vi "myRIO_BRig_Host_parse_dataBlock__v4.vi"(10 "input_dataCurrent":u16[](array[numeric]), 11 "input_dataBlock":u16[][](array[numeric])) -> (0 "BlockR_T2R_avg":dbl caption="Trials2Reward", 1 "BlockR_BTPR_avg":dbl caption="BadTrialsPostReward", 2 "BlockL_BTPR_avg":dbl caption="BadTrialsPostReward" format="%#_3g", 3 "BlockL_T2R_avg":dbl caption="Trials2Reward" format="%#_3g", 4 "BlockR_BTPR_cur":u16 caption="BadTrialsPostReward", 5 "BlockL_BTPR_cur":u16 caption="BadTrialsPostReward", 6 "BlockR_T2R_cur":u16 caption="Trials2Reward", 7 "BlockL_T2R_cur":u16 caption="Trials2Reward")   [LabVIEW 2014]
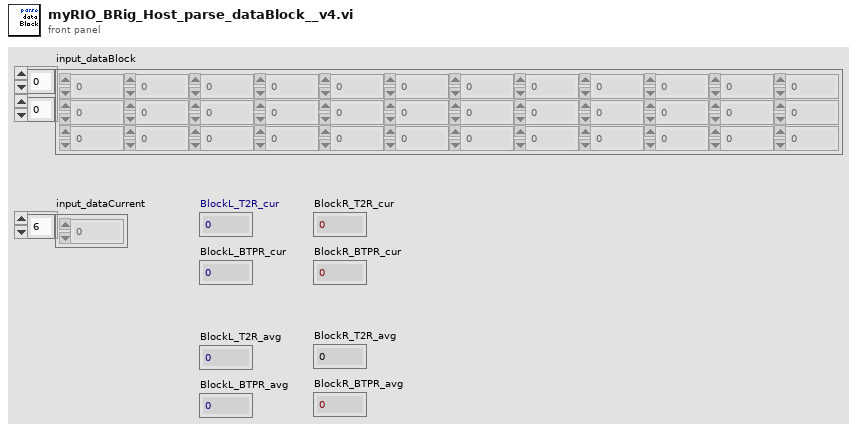
[diagram p1: front panel]
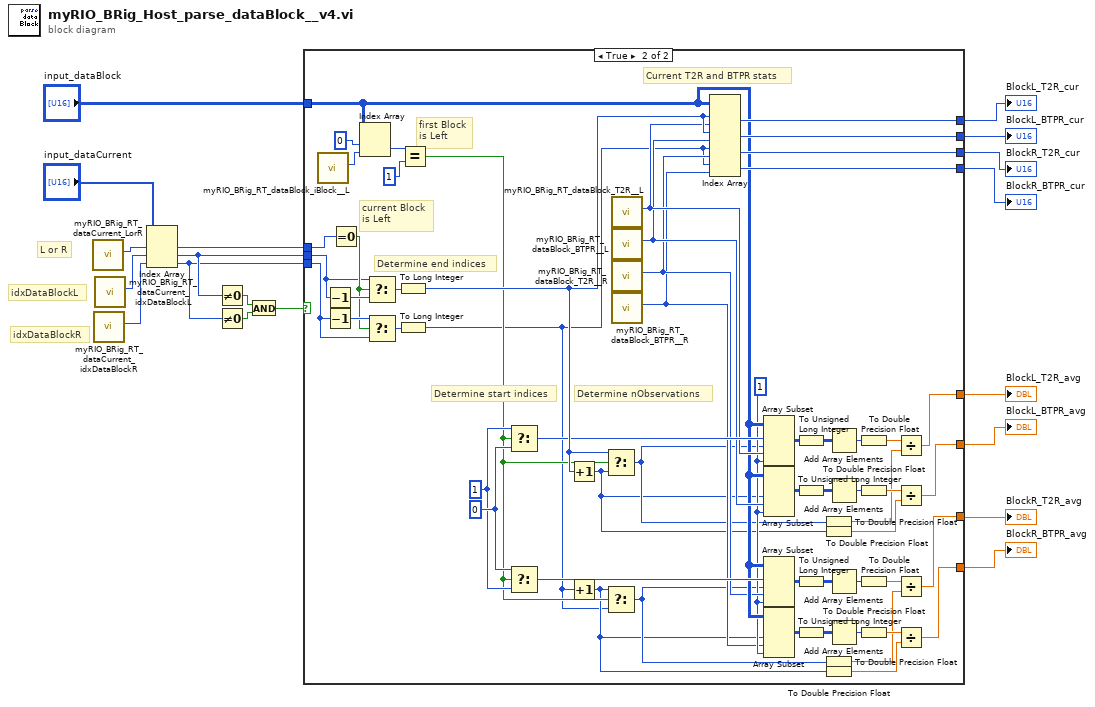
[diagram p0: block diagram]
diagram:
  # "L or R"
  # "idxDataBlockR"
  # "idxDataBlockL"
  n1 = call "myRIO_BRig_RT_dataCurrent_LorR.vi"() -> ("output_LorR"=w17:i32)  [unwired: 11 in]
  n2 = call "myRIO_BRig_RT_dataCurrent_idxDataBlockR.vi"() -> ("output_idxDataBlock__R"=w1:i32)  [unwired: 11 in]
  n3 = call "myRIO_BRig_RT_dataCurrent_idxDataBlockL.vi"() -> ("output_idxDataBlock__L"=w18:i32)  [unwired: 11 in]
  n4 = Index Array(array="input_dataCurrent", index #1=w17, index #2=w18, index #3=w1) -> (element #1=w12:u16, element #2=w11:u16, element #3=w10:u16)
  n5 = Not Equal To 0?(x=w11) -> (x != 0?=w15:bool)
  n6 = Not Equal To 0?(x=w10) -> (x != 0?=w16:bool)
  n7 = And(x=w15, y=w16) -> (x .and. y?=w14:bool)
  n8 = case shown="True" w14 {
    tunnel: "input_dataBlock" -> [_ w40]
    tunnel: w12 -> [_ w76]
    tunnel: w11 -> [_ w63]
    tunnel: w10 -> [_ w68]
    tunnel: [_ w62] -> w7
    tunnel: [_ w61] -> w6
    tunnel: [_ w50] -> w9
    tunnel: [_ w49] -> w8
    tunnel: [_ w60] -> w3
    tunnel: [_ w59] -> w2
    tunnel: [_ w47] -> w4
    tunnel: [_ w48] -> w5
    frame False {
    }
    frame True {
      w38 = 1 ("length")
      w64 = 1
      w65 = 0
      # "Current T2R and BTPR stats"
      # "Determine nObservations"
      # "Determine end indices"
      # "Determine start indices"
      # "current Block\nis Left"
      # "first Block\nis Left"
      n9 = call "myRIO_BRig_RT_dataBlock_iBlock__L.vi"() -> ("output_iBlock__L"=w75:i32)  [unwired: 11 in]
      n10 = Decrement(x=w63) -> (x-1=w71:u16)
      n11 = Decrement(x=w68) -> (x-1=w70:u16)
      n12 = Equal To 0?(x=w76) -> (x = 0?=w69:bool)
      n13 = Index Array(array=w40, index (row)=0 ("disabled index (row)"), index (col)=w75) -> (element=w73:u16)
      n14 = Select(t=w63, s=w69, f=w71) -> (s? t:f=w66:u16)
      n15 = Select(t=w70, s=w69, f=w68) -> (s? t:f=w67:u16)
      n16 = To Long Integer(number=w66) -> (32bit integer=w46:i32)
      n17 = To Long Integer(number=w67) -> (32bit integer=w20:i32)
      n18 = Equal?(x=w73, y=u16 1) -> (x = y?=w45:bool)
      n19 = Select(t=w64, s=w45, f=w65) -> (s? t:f=w44:i32)
      n20 = Select(t=w65, s=w45, f=w64) -> (s? t:f=w41:i32)
      n21 = Increment(x=w46) -> (x+1=w27:i32)
      n22 = Increment(x=w20) -> (x+1=w21:i32)
      n23 = Select(t=w46, s=w45, f=w27) -> (s? t:f=w28:i32)
      n24 = Select(t=w21, s=w45, f=w20) -> (s? t:f=w24:i32)
      n25 = call "myRIO_BRig_RT_dataBlock_T2R__L.vi"() -> ("output_T2R__L"=w43:i32)  [unwired: 11 in]
      n26 = call "myRIO_BRig_RT_dataBlock_BTPR__L.vi"() -> ("output_BTPR__L"=w42:i32)  [unwired: 11 in]
      n27 = call "myRIO_BRig_RT_dataBlock_T2R__R.vi"() -> ("output_T2R__R"=w39:i32)  [unwired: 11 in]
      n28 = call "myRIO_BRig_RT_dataBlock_BTPR__R.vi"() -> ("output_BTPR__R"=w37:i32)  [unwired: 11 in]
      n29 = Index Array(array=w40, index (row) #1=w46, index (col) #1=w43, index (row) #2=w46, index (col) #2=w42, index (row) #3=w20, index (col) #3=w39, index (row) #4=w20, index (col) #4=w37) -> (element #1=w62:u16, element #2=w61:u16, element #3=w60:u16, element #4=w59:u16)
      n30 = Array Subset(array=w40, index (row)=w44, length (row)=w28, index (col)=w43, length (col)=w38) -> (w36:u16[][])
      n31 = Array Subset(array=w40, length (row)=w27, index (col)=w42, length (col)=w38) -> (w35:u16[][])  [unwired: 1 in]
      n32 = Array Subset(array=w40, index (row)=w41, length (row)=w24, index (col)=w39, length (col)=w38) -> (w34:u16[][])
      n33 = Array Subset(array=w40, length (row)=w21, index (col)=w37, length (col)=w38) -> (w33:u16[][])  [unwired: 1 in]
      n34 = To Unsigned Long Integer(number=w36) -> (unsigned 32bit integer=w32:u32[][])
      n35 = To Unsigned Long Integer(number=w35) -> (unsigned 32bit integer=w31:u32[][])
      n36 = To Unsigned Long Integer(number=w34) -> (unsigned 32bit integer=w30:u32[][])
      n37 = To Unsigned Long Integer(number=w33) -> (unsigned 32bit integer=w29:u32[][])
      n38 = To Double Precision Float(number=w28) -> (double precision float=w26:dbl)
      n39 = To Double Precision Float(number=w27) -> (double precision float=w25:dbl)
      n40 = To Double Precision Float(number=w24) -> (double precision float=w23:dbl)
      n41 = To Double Precision Float(number=w21) -> (double precision float=w22:dbl)
      n42 = Add Array Elements(numeric array=w32) -> (sum=w58:u32)
      n43 = Add Array Elements(numeric array=w31) -> (sum=w57:u32)
      n44 = Add Array Elements(numeric array=w30) -> (sum=w56:u32)
      n45 = Add Array Elements(numeric array=w29) -> (sum=w55:u32)
      n46 = To Double Precision Float(number=w58) -> (double precision float=w54:dbl)
      n47 = To Double Precision Float(number=w57) -> (double precision float=w53:dbl)
      n48 = To Double Precision Float(number=w56) -> (double precision float=w52:dbl)
      n49 = To Double Precision Float(number=w55) -> (double precision float=w51:dbl)
      n50 = Divide(x=w54, y=w26) -> (x/y=w50:dbl)
      n51 = Divide(x=w53, y=w25) -> (x/y=w49:dbl)
      n52 = Divide(x=w52, y=w23) -> (x/y=w48:dbl)
      n53 = Divide(x=w51, y=w22) -> (x/y=w47:dbl)
    }
  }
  "BlockR_T2R_avg" <- w5
  "BlockR_BTPR_avg" <- w4
  "BlockR_T2R_cur" <- w3
  "BlockR_BTPR_cur" <- w2
  "BlockL_T2R_avg" <- w9
  "BlockL_BTPR_avg" <- w8
  "BlockL_T2R_cur" <- w7
  "BlockL_BTPR_cur" <- w6
